vi "Configure Q-Switch Frequency.vi"(8 "error in (no error)":errorcluster, 10 "frequency, Hz":dbl, 11 "Lotis in":refnum<class "PL Lotis TII LS.lvclass">) -> (0 "error out":errorcluster, 3 "Lotis out":refnum<class "PL Lotis TII LS.lvclass">)   [LabVIEW 2015, in "PL Lotis TII LS.lvclass"]
doc: "Configures Q-Switch frequency."
uses:
  PL Lotis TII LS.lvclass
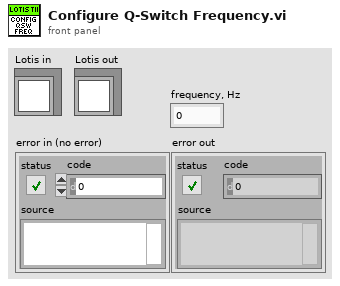
[diagram p1: front panel]
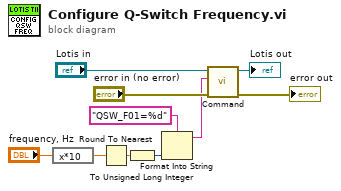
[diagram p0: block diagram]
diagram:
  n1 = expression code="x*10"("frequency, Hz") -> (w3:dbl)
  n2 = Round To Nearest(number=w3) -> (nearest integer value=w2:dbl)
  n3 = To Unsigned Long Integer(number=w2) -> (unsigned 32bit integer=w1:u32)
  n4 = Format Into String(format string="QSW_F01=%d" ("command"), w1) -> (resulting string=w5:string)  [unwired: 2 in, 1 out]
  n5 = call "Command.vi"("error in (no error)"="error in (no error)", "command"=w5, "Lotis in"="Lotis in") -> ("error out"=→"error out":errorcluster, "Lotis out"=→"Lotis out":refnum<class "PL Lotis TII LS.lvclass">)  [unwired: 6 in, 1 out]
